vi "Detect Multiple.vi"   [LabVIEW 2020, in "feature_detection.lvlib" / "QR Code Detector.lvclass"]
doc: "Detect multiple QR Codes in an image."
uses:
  QR Code Detector.lvclass
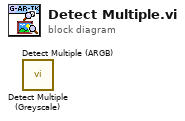
[diagram p0: block diagram]
diagram:
  n1 = call "Detect Multiple (Greyscale).vi"() -> ()  [unwired: 7 in, 5 out]
  n2 = call "Detect Multiple (ARGB).vi"() -> ()  [unwired: 7 in, 5 out]
